vi "Get Subtype Description.vi"(8 "error in (no error)":errorcluster, 11 "Numeric Assertion in":refnum<class "Numeric Assertion.lvclass">) -> (0 "error out":errorcluster, 2 "Subtype Description":string, 3 "Numeric Assertion out":refnum<class "Numeric Assertion.lvclass">)   [LabVIEW 2020, in "MacroAssert.lvlib" / "Numeric Assertion.lvclass"]
doc: "Gets the subtype description for <B>Step in</B>, which describes what the step's subtype does specifically."
uses:
  Numeric Assertion.lvclass
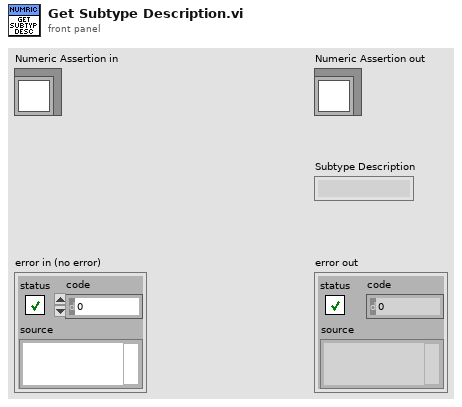
[diagram p1: front panel]
types:
  T1 = typedef "MacroAssert.lvlib/Numeric Assertion.lvclass/Numeric Assertion Type.ctl" = enum16{"Numeric Ctl Value", "Array Ctl Size", "Ctl Width Property", "Ctl Height Property", "VI Width", "VI Height", "Window Width", "Window Height", "Window Scale", "Number of Displays", "Highest Display Scale"}
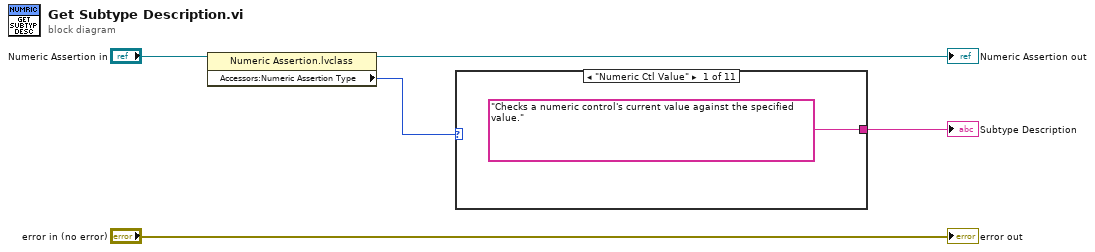
[diagram p0: block diagram]
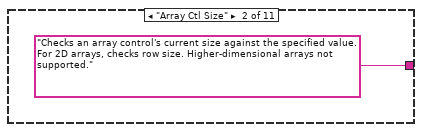
[diagram p2: hidden frame]
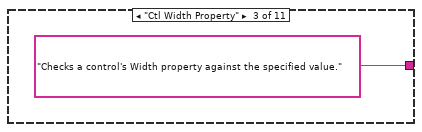
[diagram p3: hidden frame]
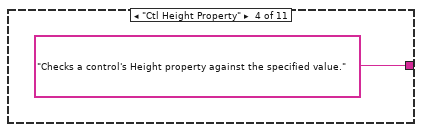
[diagram p4: hidden frame]
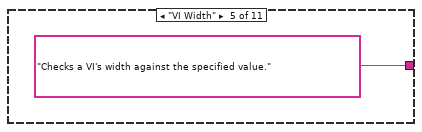
[diagram p5: hidden frame]
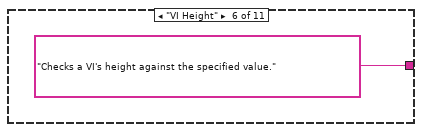
[diagram p6: hidden frame]
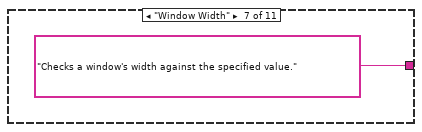
[diagram p7: hidden frame]
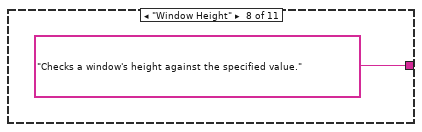
[diagram p8: hidden frame]
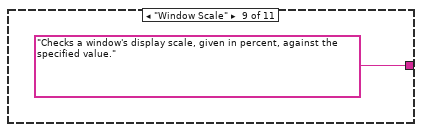
[diagram p9: hidden frame]
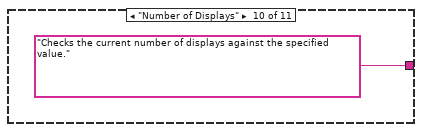
[diagram p10: hidden frame]
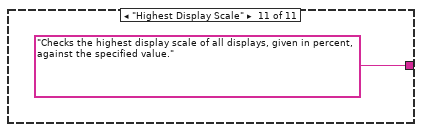
[diagram p11: hidden frame]
diagram:
  n1 = property class="Numeric Assertion.lvclass"(reference="Numeric Assertion in") -> (reference out=→"Numeric Assertion out":refnum<class "Numeric Assertion.lvclass">, "Accessors:Numeric Assertion Type"=w5:T1)  [unwired: 1 in, 1 out]
  n2 = case shown="\"Numeric Ctl Value\"" w5 {
    tunnel: ["Checks a numeric control's current value against the specified value." "Checks an array control's current size against the specified value. For 2D arrays, checks row size. Higher-dimensional arrays not supported." "Checks a control's Width property against the specified value." "Checks a control's Height property against the specified value." "Checks a VI's width against the specified value." "Checks a VI's height against the specified value." "Checks a window's width against the specified value." "Checks a window's height against the specified value." "Checks a window's display scale, given in percent, against the specified value." "Checks the current number of displays against the specified value." "Checks the highest display scale of all displays, given in percent, against the specified value."] -> w1
    frame "Numeric Ctl Value" {
    }
    frame "Array Ctl Size" {
    }
    frame "Ctl Width Property" {
    }
    frame "Ctl Height Property" {
    }
    frame "VI Width" {
    }
    frame "VI Height" {
    }
    frame "Window Width" {
    }
    frame "Window Height" {
    }
    frame "Window Scale" {
    }
    frame "Number of Displays" {
    }
    frame "Highest Display Scale" {
    }
  }
  "Subtype Description" <- w1
  "error out" <- "error in (no error)"
